vi "get desired keys.vi"(8 "error in":errorcluster, 11 "ExampleStateMachine configuration in":refnum<class "ExampleStateMachine configuration.lvclass">) -> (0 "error out":errorcluster, 2 "desired keys":string[](array[string]), 3 "ExampleStateMachine configuration out":refnum<class "ExampleStateMachine configuration.lvclass">)   [LabVIEW 2017, in "ExampleStateMachine configuration.lvclass"]
uses:
  ExampleStateMachine configuration.lvclass
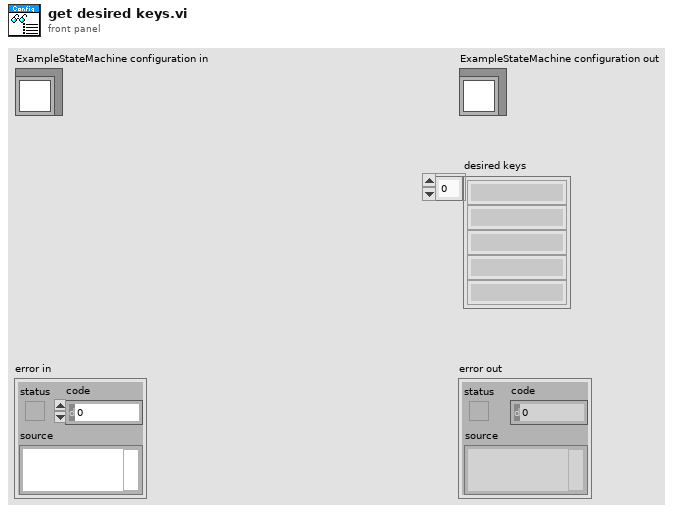
[diagram p1: front panel]
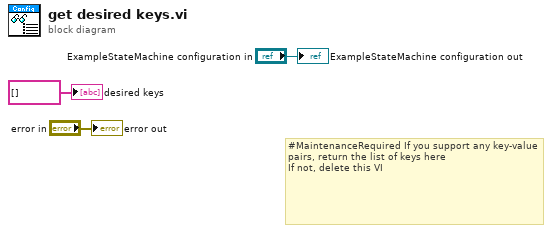
[diagram p0: block diagram]
diagram:
  # "#MaintenanceRequired If you support any key-value pairs, return the list of keys here\nIf not, delete this VI"
  "error out" <- "error in"
  "ExampleStateMachine configuration out" <- "ExampleStateMachine configuration in"
  "desired keys" <- string[] [] ("desired keys")
